vi "Launch NS.vi"(8 "error in":errorcluster, 11 "MiniGUI in":refnum<class "MiniGUI.lvclass">) -> (0 "error out":errorcluster, 3 "MiniGUI out":refnum<class "MiniGUI.lvclass">)   [LabVIEW 2019]
uses:
  <vilib>/ActorFramework/Actor/Actor.lvclass
  Network Stream/Network Stream.lvclass
  MiniGUI Messages/Receive Dataset Msg/Receive Dataset Msg.lvclass
  MiniGUI Messages/Receive Connection Msg/Receive Connection Msg.lvclass
  MiniGUI.lvclass
  C:/Program Files (x86)/National Instruments/LabVIEW 2019/vi.lib/MGI/Panel Manager/Panel Actor/Panel Actor/Panel Actor.lvclass
  C:/Program Files (x86)/National Instruments/LabVIEW 2019/vi.lib/MGI/Monitored Actor/Monitored Actor/Monitored Actor/Monitored Actor.lvclass
  C:/Program Files (x86)/National Instruments/LabVIEW 2019/vi.lib/ActorFramework/Actor/Actor.lvclass
  C:/Working Copy/trunk/Modified Cobra Jung/Cobra/Cobra AF/Network Stream/Network Stream Messages/NS Connection Msg/NS Connection Msg.lvclass
  C:/Program Files (x86)/National Instruments/LabVIEW 2019/vi.lib/ActorFramework/Message/Message.lvclass
  C:/Working Copy/trunk/Modified Cobra Jung/Cobra/Cobra AF/Network Stream/Network Stream Messages/Dataset Msg/Dataset Msg.lvclass
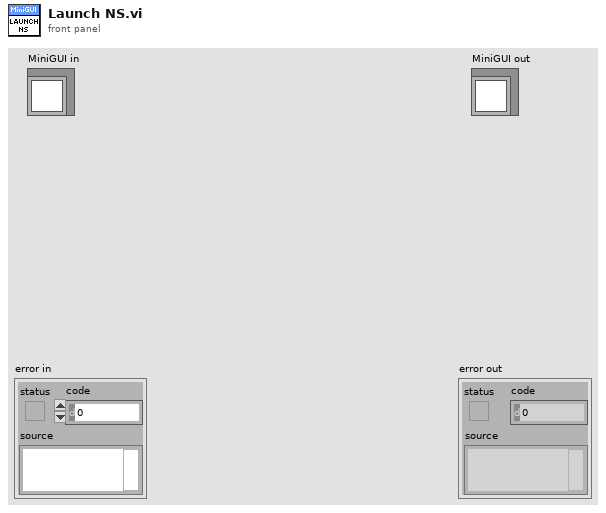
[diagram p1: front panel]
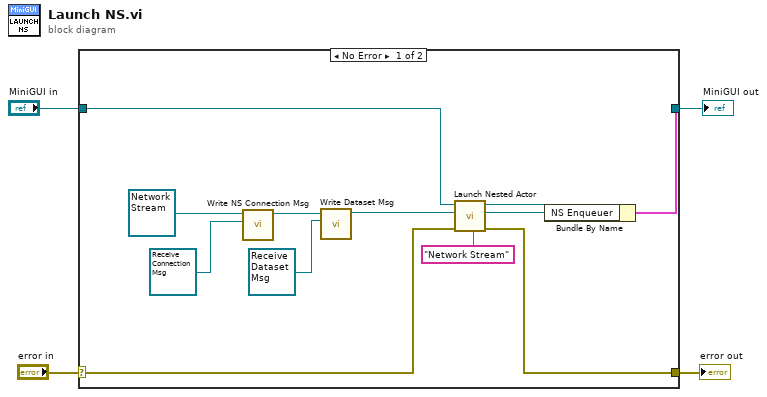
[diagram p0: block diagram]
diagram:
  n1 = case shown="No Error" "error in" {
    selector: "error in" -> [w14 w18]
    tunnel: [w13 w18] -> w3
    tunnel: [w10 w17] -> w1
    tunnel: "MiniGUI in" -> [w12 w17]
    frame No Error {
      n2 = call "Write NS Connection Msg.vi"("GUI.lvlib:Network Stream.lvlib:NS Connection Msg.lvclass"=refnum<class "Receive Connection Msg.lvclass"> refnum ("MiniGUI.lvlib:Receive Connection Msg.lvclass"), "Network Stream in"=refnum<class "Network Stream.lvclass"> refnum ("Network Stream.lvlib:Network Stream.lvclass")) -> ("Network Stream out"=w8:refnum<class "Network Stream.lvclass">)  [unwired: 9 in]
      n3 = call "Write Dataset Msg.vi"("GUI.lvlib:Network Stream.lvlib:Dataset Msg.lvclass"=refnum<class "Receive Dataset Msg.lvclass"> refnum ("MiniGUI.lvlib:Receive Dataset Msg.lvclass"), "Network Stream in"=w8) -> ("Network Stream out"=w7:refnum<class "Network Stream.lvclass">)  [unwired: 9 in]
      n4 = call <vilib>:"Launch Nested Actor.vi"("Debug Alias"="Network Stream", "error in (no error)"=w14, "Nested Actor"=w7, "Caller Actor in"=w12) -> ("error out"=w13:errorcluster, "Nested Actor's Enqueuer"=w16:refnum<class "Message Enqueuer.lvclass">, "Caller Actor out"=w11:refnum<class "MiniGUI.lvclass">)  [unwired: 5 in]
      n5 = Bundle By Name(cluster=w11, "NS Enqueuer"=w16) -> (w10:cluster{})
    }
    frame Error {
    }
  }
  "error out" <- w3
  "MiniGUI out" <- w1
